vi "Pre Launch Init.vi"(11 "Sensor View in":refnum<class "Sensor View.lvclass">) -> (0 "error out":errorcluster, 3 "Sensor View out":refnum<class "Sensor View.lvclass">)   [LabVIEW 2013, in "Sensor View.lvlib" / "Sensor View.lvclass"]
doc: "(<B>Filename</B>: Actor Framework.lvlib:Actor.lvclass:Pre Launch Init.vi)\n\nDefines behavior that occurs after the Launch Actor method is invoked but before the actor's Actor Core method begins running.\n\nThe Pre Launch Init method is guaranteed to finish before the Launch Actor method returns to its caller and before the actor itself receives any messages. Any references that the Pre Launch Init method obtains are guaranteed to have the same lifetime as the actor itself. Any errors that the Pre Launch Init method returns will abort the launch.\n\nBy default, this method does nothing. A descendant class may override it to define behavior."
uses:
  Sensor View.lvclass
  Sensor View.lvclass/Sensor View.ctl
  <vilib>/ActorFrameworkMVC/View Actor/View Actor.lvclass
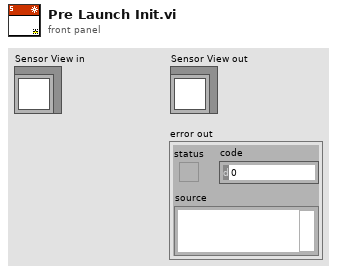
[diagram p1: front panel]
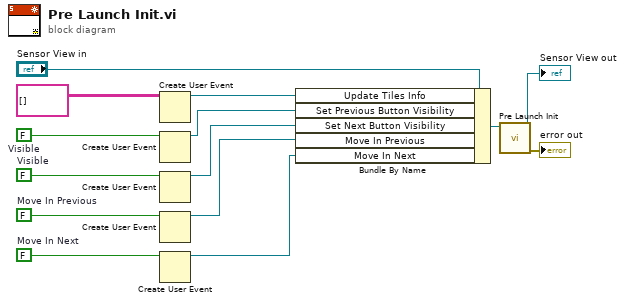
[diagram p0: block diagram]
diagram:
  w3 = FALSE  # Move In Next
  w4 = FALSE  # Move In Previous
  w10 = FALSE  # Visible
  w11 = FALSE  # Visible
  n1 = Create User Event(user event datatype=string[][] [] ("Tiles Info")) -> (user event=w6:refnum<user-event>)  [unwired: 1 in, 1 out]
  n2 = Create User Event(user event datatype=w11) -> (user event=w9:refnum<user-event>)  [unwired: 1 in, 1 out]
  n3 = Create User Event(user event datatype=w10) -> (user event=w8:refnum<user-event>)  [unwired: 1 in, 1 out]
  n4 = Create User Event(user event datatype=w4) -> (user event=w2:refnum<user-event>)  [unwired: 1 in, 1 out]
  n5 = Create User Event(user event datatype=w3) -> (user event=w1:refnum<user-event>)  [unwired: 1 in, 1 out]
  n6 = Bundle By Name(cluster="Sensor View in", "Update Tiles Info"=w6, "Set Previous Button Visibility"=w9, "Set Next Button Visibility"=w8, "Move In Previous"=w2, "Move In Next"=w1) -> (w12:refnum<class "Sensor View.lvclass">)
  n7 = call-parent "Pre Launch Init.vi"("Actor in"=w12) -> ("error out"=→"error out":errorcluster, "Actor out"=→"Sensor View out":refnum<class "Sensor View.lvclass">)  [unwired: 9 in]
